vi "Coms Hardware Driver Main.vi"(8 "error IN":errorcluster, 11 "Instance Details":T1) -> ()   [LabVIEW 2014]
uses:
  Aircraft Data Router/Controls/Known Aircraft.ctl
  Controls/Coms Driver Interface.ctl
  Telemetry/Controls/Telemetry Connection Type.ctl
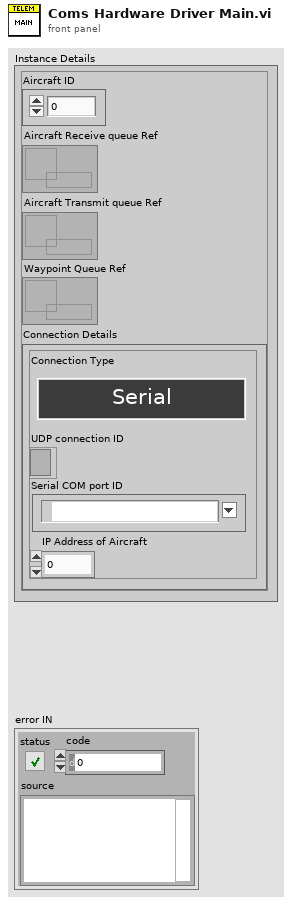
[diagram p1: front panel]
types:
  T1 = typedef "Known Aircraft.ctl" = cluster{"Aircraft ID":u8, "Aircraft Receive queue Ref":refnum<queue>, "Aircraft Transmit queue Ref":refnum<queue>, "Waypoint Queue Ref":refnum<queue>, "Connection Details":T2}
  T2 = typedef "Coms Driver Interface.ctl" = cluster{"Connection Type":T3, "UDP connection ID":refnum<k16>, "Serial COM port ID":refnum<visa-resource-name>, "IP Address of Aircraft":u32}
  T3 = typedef "Telemetry Connection Type.ctl" = enum16{"Serial", "UDP", "TCP"}
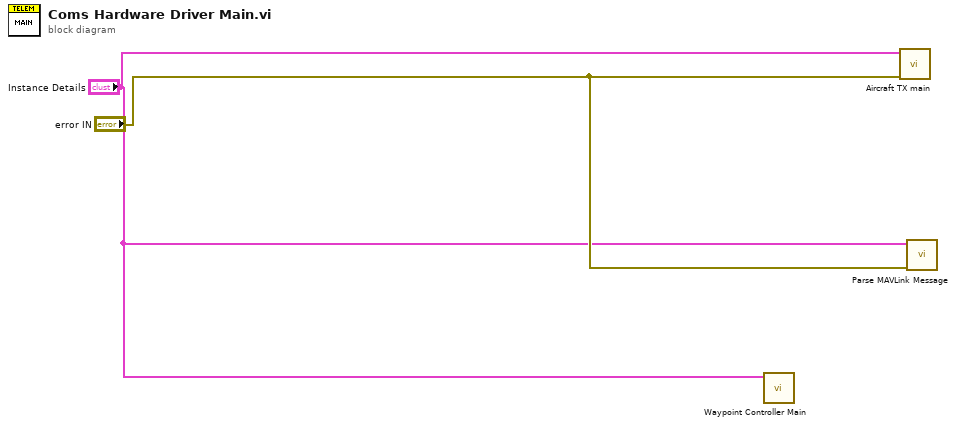
[diagram p0: block diagram]
diagram:
  n1 = call "Waypoint Controller Main.vi"("Instance Details"="Instance Details") -> ()  [unwired: 11 in]
  n2 = call "Aircraft TX main.vi"("Error In"="error IN", "Instance Details"="Instance Details") -> ()  [unwired: 10 in]
  n3 = call "Parse MAVLink Message.vi"("error in (no error)"="error IN", "Instance Details"="Instance Details") -> ()  [unwired: 10 in]
